vi "Create Error.vi"(4 "Stack Trace":string, 5 "Test Case in":refnum<class "Test Case.lvclass">, 6 "Message":string, 7 "Type":string, 8 "error in (no error)":errorcluster, 9 "Time":dbl, 10 "Classname":string, 11 "Name":string) -> (0 "error out":errorcluster, 3 "Test Case":refnum<class "Test Case.lvclass">)   [LabVIEW 2013, in "JUnit XML.lvlib" / "Test Case.lvclass"]
uses:
  Test Case.lvclass
  Test Result.ctl
  Test Case.lvclass/Test Case.ctl
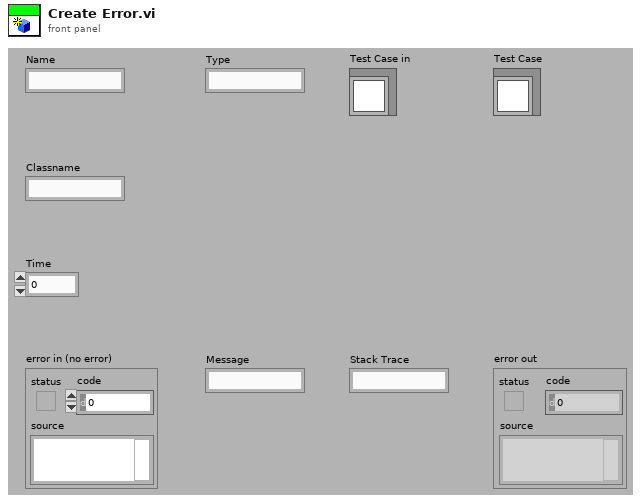
[diagram p1: front panel]
types:
  T1 = typedef "JUnit XML.lvlib/Test Case.lvclass/Test Result.ctl" = enum16{"Success", "Failure", "Error", "Skipped"}
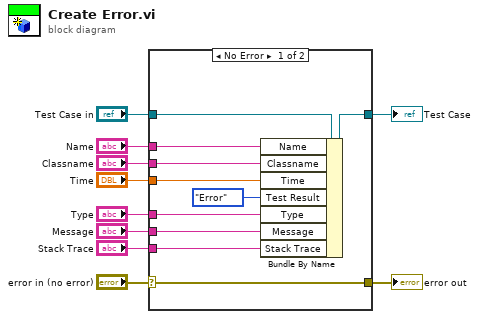
[diagram p0: block diagram]
diagram:
  n1 = case shown="No Error" "error in (no error)" {
    selector: "error in (no error)" -> [w20 w22]
    tunnel: [w20 w22] -> w9
    tunnel: [w18 w21] -> w7
    tunnel: "Test Case in" -> [w19 w21]
    tunnel: "Name" -> [w17 _]
    tunnel: "Classname" -> [w16 _]
    tunnel: "Time" -> [w15 _]
    tunnel: "Type" -> [w13 _]
    tunnel: "Message" -> [w12 _]
    tunnel: "Stack Trace" -> [w11 _]
    frame No Error {
      n2 = Bundle By Name(cluster=w19, "Name"=w17, "Classname"=w16, "Time"=w15, "Test Result"=Test_Result."Error", "Type"=w13, "Message"=w12, "Stack Trace"=w11) -> (w18:refnum<class "Test Case.lvclass">)
    }
    frame Error {
    }
  }
  "error out" <- w9
  "Test Case" <- w7
